vi "virtual.vi"(1 "Pitch":i32(slide) scale=-90.0..90.0, 2 "Roll":i32(slide) scale=90.0..-90.0) -> (0 "Virtual Horizont":picture)   [LabVIEW 2009]
uses:
  Rotate.llb/rotate 24bit.vi
panel:
  in  "stop":bool
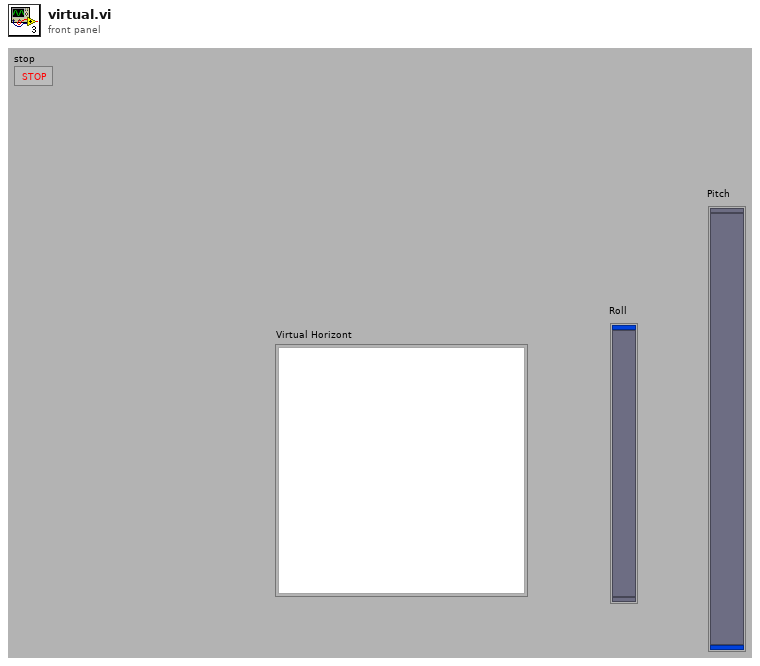
[diagram p1: front panel]
types:
  T1 = cluster{"left":i16, "top":i16, "right":i16, "bottom":i16}
  T2 = typedef "imagedata.ctl" = cluster{"image type":i32, "image depth":i32, "image":u8[], "mask":u8[], "colors":u32[], "Rectangle":cluster{"left":i16, "top":i16, "right":i16, "bottom":i16}}
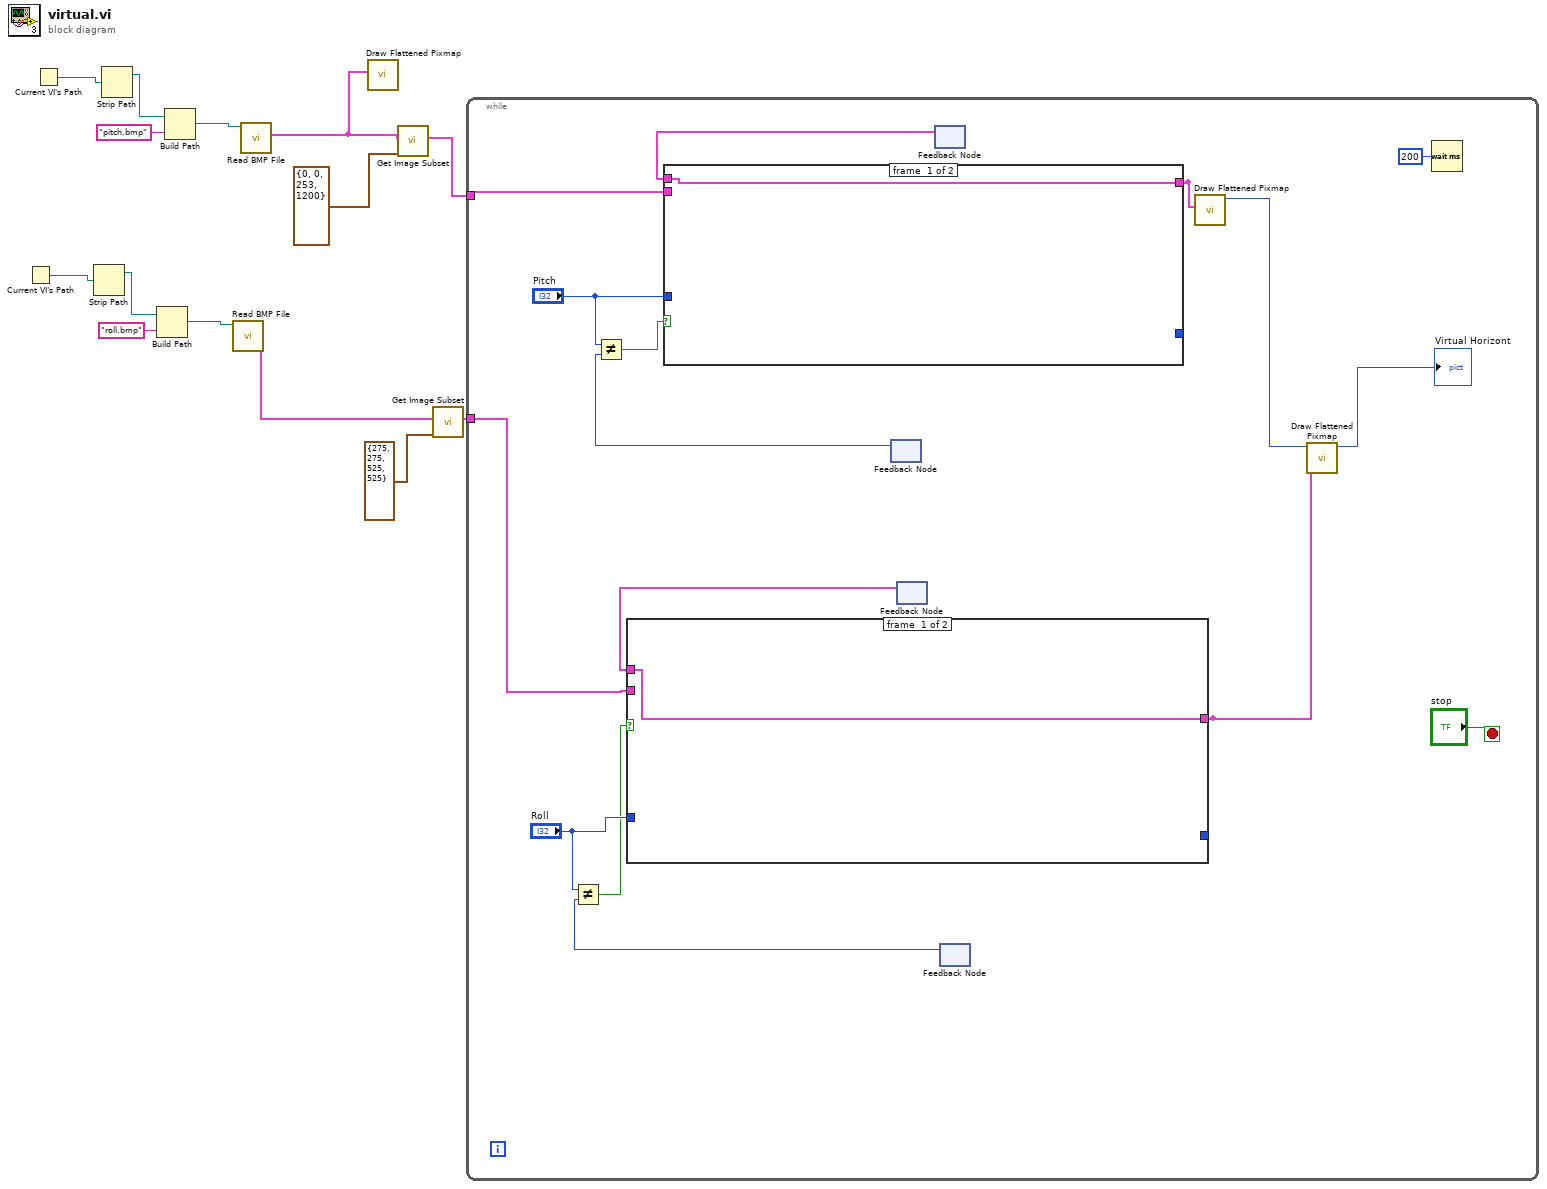
[diagram p0: block diagram]
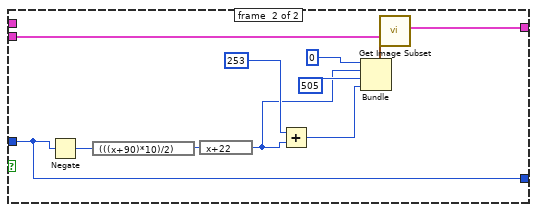
[diagram p2: hidden frame]
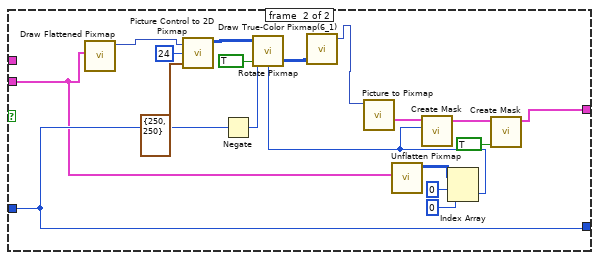
[diagram p3: hidden frame]
diagram:
  n1 = Current VI's Path() -> (path=w3:path)
  n2 = Current VI's Path() -> (path=w12:path)
  n3 = Strip Path(path=w3) -> (stripped path=w2:path)  [unwired: 1 out]
  n4 = Strip Path(path=w12) -> (stripped path=w11:path)  [unwired: 1 out]
  n5 = Build Path(base path=w2, name or relative path="roll.bmp") -> (appended path=w4:path)
  n6 = Build Path(base path=w11, name or relative path="pitch.bmp") -> (appended path=w13:path)
  n7 = call <vilib>:"Read BMP File.vi"("path to BMP file"=w4) -> ("image data"=w1:T2)  [unwired: 1 in, 9 out]
  n8 = call <vilib>:"Read BMP File.vi"("path to BMP file"=w13) -> ("image data"=w8:T2)  [unwired: 1 in, 9 out]
  n9 = call <vilib>:"Draw Flattened Pixmap.vi"("image data"=w8) -> ()  [unwired: 1 in, 8 out]
  n10 = call <vilib>:"Get Image Subset.vi"("subset rect"=T1 {"left"=0, "top"=0, "right"=253, "bottom"=1200}, "image data"=w8) -> ("image subset"=w9:T2)  [unwired: 5 out]
  n11 = call <vilib>:"Get Image Subset.vi"("subset rect"=T1 {"left"=275, "top"=275, "right"=525, "bottom"=525}, "image data"=w1) -> ("image subset"=w6:T2)  [unwired: 5 out]
  n12 = while {
    tunnel: w9 -> [w32]
    tunnel: w6 -> [w23]
    stop <- "stop" stop-if-true
    n13 = feedback #1() -> (w18:i32)  [unwired: 1 out]
    n14 = Not Equal?(x="Pitch", y=w18) -> (x != y?=w21:bool)
    n15 = feedback #2() -> (w24:T2)  [unwired: 1 out]
    n16 = feedback #3() -> (w16:T2)  [unwired: 1 out]
    n17 = case shown="False" w21 {
      tunnel: w32 -> [_ w44]
      tunnel: "Pitch" -> [_ w34]
      tunnel: [w33 w35] -> w17
      tunnel: [_ w34] -> w19
      tunnel: w16 -> [w33 _]
      frame #0 {
      }
      frame #1 {
        n18 = Negate(x=w34) -> (-x=w36:i32)
        n19 = expression code="(((x+90)*10)/2)"(w36) -> (w37:i32)
        n20 = expression code="x+22"(w37) -> (w38:i32)
        n21 = Add(x=253, y=w38) -> (x+y=w39:i32)
        n22 = Bundle(0, w38, 505, w39) -> (w43:cluster{i32, i32, i32, i32})  [unwired: 1 out]
        n23 = call <vilib>:"Get Image Subset.vi"("subset rect"=w43, "image data"=w44) -> ("image subset"=w35:T2)  [unwired: 5 out]
      }
    }
    n24 = feedback #4() -> (w29:i32)  [unwired: 1 out]
    n25 = Not Equal?(x="Roll", y=w29) -> (x != y?=w27:bool)
    n26 = case shown="True" w27 {
      tunnel: "Roll" -> [_ w49]
      tunnel: w23 -> [_ w48]
      tunnel: [_ w49] -> w30
      tunnel: [w45 w46] -> w25
      tunnel: w24 -> [w45 _]
      frame #0 {
      }
      frame #1 {
        n27 = call <vilib>:"Draw Flattened Pixmap.vi"("image data"=w48) -> ("new picture"=w47:picture)  [unwired: 1 in, 7 out]
        n28 = call "Picture Control to 2D Pixmap.vi"("Picture"=w47, "image depth"=u8 24, "Draw Area Size"=cluster{"Width":u32, "Height":u32} {"Width"=250, "Height"=250}) -> ("24-bit"=w54:u32[][])  [unwired: 4 out]
        n29 = Negate(x=w49) -> (-x=w63:i32)
        n30 = call <vilib>:"Unflatten Pixmap.vi"("image data"=w48) -> ("24-bit pixmap"=w52:u32[][])  [unwired: 10 out]
        n31 = Index Array(array=w52, index (row)=0, index (col)=0 ("disabled index (col)")) -> (element=w60:u32)
        n32 = call-poly "Rotate Pixmap.vi"("Color Table Index of Fill Color"=w60, "Maintain Center Position?"=TRUE, "Rotation Angle (degrees)"=w63, "Pixmap"=w54) -> ("Rotated Pixmap"=w58:u32[][])
        n33 = call <vilib>:"Draw True-Color Pixmap(6_1).vi"("data (RGB format)"=w58) -> ("new picture"=w51:picture)  [unwired: 2 in, 6 out]
        n34 = call <vilib>:"Picture to Pixmap.vi"("picture"=w51) -> ("image data"=w59:T2)  [unwired: 3 in, 7 out]
        n35 = call <vilib>:"Create Mask.vi"("Mask Color (Black)"=w60, "image data"=w59) -> ("image data"=w61:T2)  [unwired: 2 in, 7 out]
        n36 = call <vilib>:"Create Mask.vi"("Combine Masks? (F)"=TRUE, "image data"=w61) -> ("image data"=w46:T2)  [unwired: 2 in, 7 out]
      }
    }
    n37 = call <vilib>:"Draw Flattened Pixmap.vi"("image data"=w17) -> ("new picture"=w22:picture)  [unwired: 1 in, 7 out]
    n38 = call <vilib>:"Draw Flattened Pixmap.vi"("image data"=w25, "picture"=w22) -> ("new picture"=→"Virtual Horizont":picture)  [unwired: 7 out]
    n39 = Wait (ms)(milliseconds to wait=u32 200) -> ()  [unwired: 1 out]
  }
